vi "Destroy.vi"(8 "error in (no error)":errorcluster, 11 "Bus in":refnum<class "Bus.lvclass">) -> (0 "error out":errorcluster, 3 "Bus out":refnum<class "Bus.lvclass">)   [LabVIEW 2014]
uses:
  Bus.lvclass
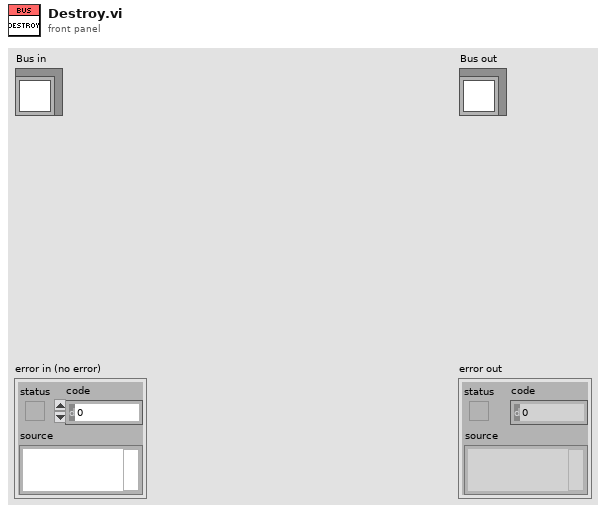
[diagram p1: front panel]
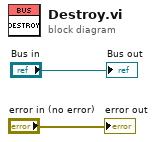
[diagram p0: block diagram]
diagram:
  "error out" <- "error in (no error)"
  "Bus out" <- "Bus in"
